vi "labview_client(not_used).vi"() -> ()   [LabVIEW 2018]
doc: "You can use the System Exec VI to call command line utilities that return standard output to the command shell. You also can call interactive applications that you intend to launch using System Exec, but interact with using the UI of the executable."
panel:
  out "standard output":string
  in  "Stop Button":bool
  out "standard error":string
  out "return code":i32
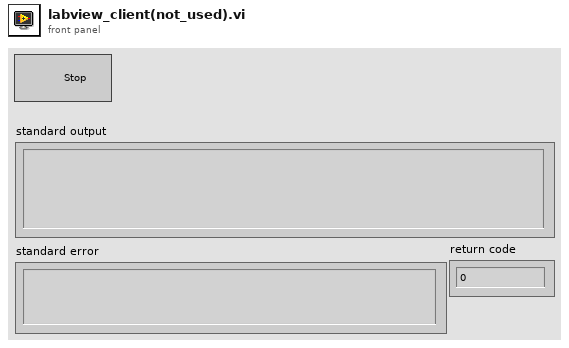
[diagram p1: front panel]
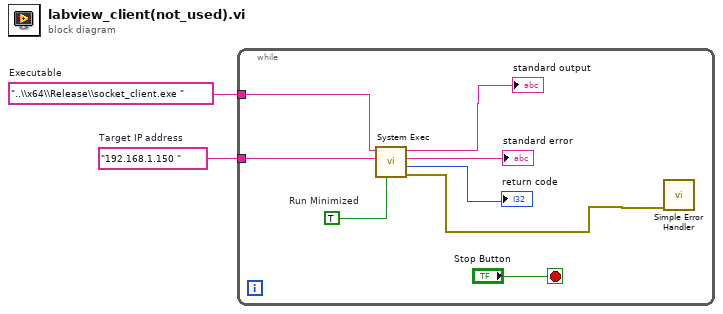
[diagram p0: block diagram]
diagram:
  w2 = "..\\x64\\Release\\socket_client.exe "  # Executable
  w1 = "192.168.1.150 "  # Target IP address
  n1 = while {
    tunnel: w1 -> [w8]
    tunnel: w2 -> [w7]
    stop <- "Stop Button" stop-if-true
    w9 = TRUE  # Run Minimized
    n2 = call <vilib>:"System Exec.vi"("run minimized? (F)"=w9, "standard input"=w8, "command line"=w7) -> ("error out"=w3:errorcluster, "return code"=→"return code":i32, "standard error"=→"standard error":string, "standard output"=→"standard output":string)  [unwired: 5 in]
    n3 = call <vilib>:"Simple Error Handler.vi"("error in (no error)"=w3) -> ()  [unwired: 2 in, 7 out]
  }
